vi "IMMU - Get Gyro Offsets.vi"(8 "error in (no error)":errorcluster, 11 "I2C Ref In":T1={"myRIO Reference"={"myRIO Model"=enum."Unknown", "myRIO Hardware Reference"={"Generic FPGA Reference"=refnum, "Allow multiple opens"=FALSE}}, "I2C Channels Enum"=enum."Not Connected", "I2C Configuration"={"I2C Transfer Rate"=enum."Fast mode (400 kbps)"}}) -> (0 "error out":errorcluster, 2 "Output Offset Array (int)":i16[](array[numeric]), 3 "I2C Ref Out":T1={"myRIO Reference"={"myRIO Model"=enum."Unknown", "myRIO Hardware Reference"={"Generic FPGA Reference"=refnum, "Allow multiple opens"=FALSE}}, "I2C Channels Enum"=enum."Not Connected", "I2C Configuration"={"I2C Transfer Rate"=enum."Fast mode (400 kbps)"}})   [LabVIEW 2021]
uses:
  <vilib>/myRIO/Instrument Drivers/Onboard IO/I2C/typedefs/I2C Reference.ctl
  <vilib>/myRIO/Common/Instrument Driver Framework/Utilities/typedefs/myRIO Generic Hardware Reference.ctl
  <vilib>/myRIO/Common/Instrument Driver Framework/Utilities/typedefs/Hardware Version Enum.ctl
  <vilib>/myRIO/Common/Instrument Driver Framework/Utilities/typedefs/myRIO v1.0 Reference.ctl
  <vilib>/myRIO/Common/Instrument Driver Framework/Utilities/typedefs/Generic FPGA Reference.ctl
  <vilib>/myRIO/Common/Instrument Driver Framework/myRIO v1.0/I2C/typedefs/I2C Channels Enum.ctl
  <vilib>/myRIO/Instrument Drivers/Onboard IO/I2C/typedefs/I2C Configuration.ctl
  <vilib>/myRIO/Instrument Drivers/Onboard IO/I2C/typedefs/I2C Transfer Rate.ctl
  <vilib>/Platform/TimedLoop/XDataNode/timing_clust.ctl
  <vilib>/Platform/TimedLoop/XDataNode/nitl_modes.ctl
  <vilib>/Platform/TimedLoop/XDataNode/wakeup.ctl
  <vilib>/Utility/error.llb/Error Cluster From Error Code.vi
  <vilib>/myRIO/Common/Instrument Driver Framework/myRIO v1.0/I2C/vis/myRIO v1.0 Write I2C.vi
  <vilib>/myRIO/Common/Instrument Driver Framework/myRIO v1.0/I2C/vis/myRIO v1.0 Read I2C.vi
  <vilib>/platform/TimedLoop/XDataNode/XDataNode.xnode
  <vilib>/Platform/TimedLoop/XDataNode/XDNodeRunTimeDep.lvlib
  <vilib>/myRIO/Instrument Drivers/Onboard IO/I2C/I2C.lvlib
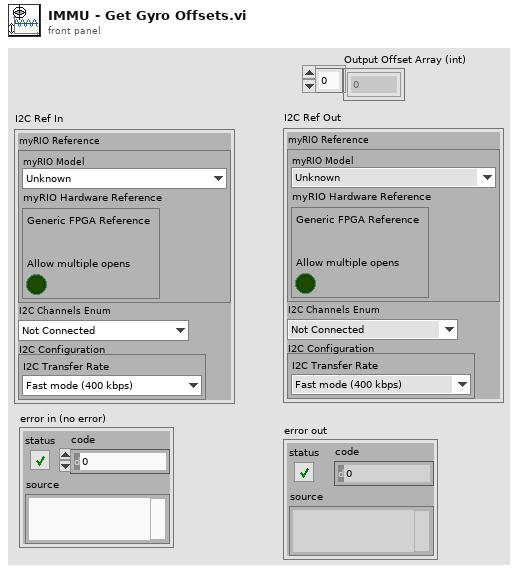
[diagram p1: front panel]
types:
  T1 = typedef "I2C.lvlib/I2C Reference.ctl" = cluster{"myRIO Reference":T2, "I2C Channels Enum":T6, "I2C Configuration":T7}
  T2 = typedef "myRIO Generic Hardware Reference.ctl" = cluster{"myRIO Model":T3, "myRIO Hardware Reference":T4}
  T3 = typedef "Hardware Version Enum.ctl" = enum16{"Unknown", "myRIO-1900", "myRIO-1950", "roboRIO", "NI ELVIS RIO CM", "ELVIS III"}
  T4 = typedef "myRIO v1.0 Reference.ctl" = cluster{"Generic FPGA Reference":T5, "Allow multiple opens":bool}
  T5 = typedef "Generic FPGA Reference.ctl" = refnum<k20>
  T6 = typedef "I2C Channels Enum.ctl" = enum16{"Not Connected", "A/I2C", "B/I2C", "I2C/I2C"}
  T7 = typedef "I2C.lvlib/I2C Configuration.ctl" = cluster{"I2C Transfer Rate":T8}
  T8 = typedef "I2C.lvlib/I2C Transfer Rate.ctl" = enum16{"Standard mode (100 kbps)", "Fast mode (400 kbps)"}
  T9 = typedef "XDNodeRunTimeDep.lvlib/timing_clust.ctl" = cluster{"Expected End [f-1]":u64, "Actual End [f-1]":u64, "Finished Late? [f-1]":bool, "Expected End [i-1]":u64, "Actual End [i-1]":u64, "Finished Late? [i-1]":bool, "Expected Start [i]":u64, "Actual Start [i]":u64, "Expected Start [f]":u64, "Actual Start [f]":u64, "Source Name":string, "Structure Name":string, "Period":i64, "Deadline":i64, "Offset":i64, "Start":i64, "Priority":i32, "Timeout":i32, "Mode":T10, "Wakeup Reason":T11, "Error":errorcluster, "Source Type":string, "Secondary Source Type":string, "Global End Time":u64, "Global Start Time":u64, "Frame Duration":u64, "Iteration Duration":u64, "Assigned CPU":i32, "I/O Scan Engine Mode":u32}
  T10 = typedef "XDNodeRunTimeDep.lvlib/nitl_modes.ctl" = enum32{"No Change", "Process missed periods, maintain original phase", "Discard missed periods, maintain original phase", "Process missed periods, ignore original phase", "Discard missed periods, ignore original phase"}
  T11 = typedef "XDNodeRunTimeDep.lvlib/wakeup.ctl" = enum32{"Normal", "Aborted", "Asynchronous wakeup", "Timing source error", "Timed loop error", "Timeout"}
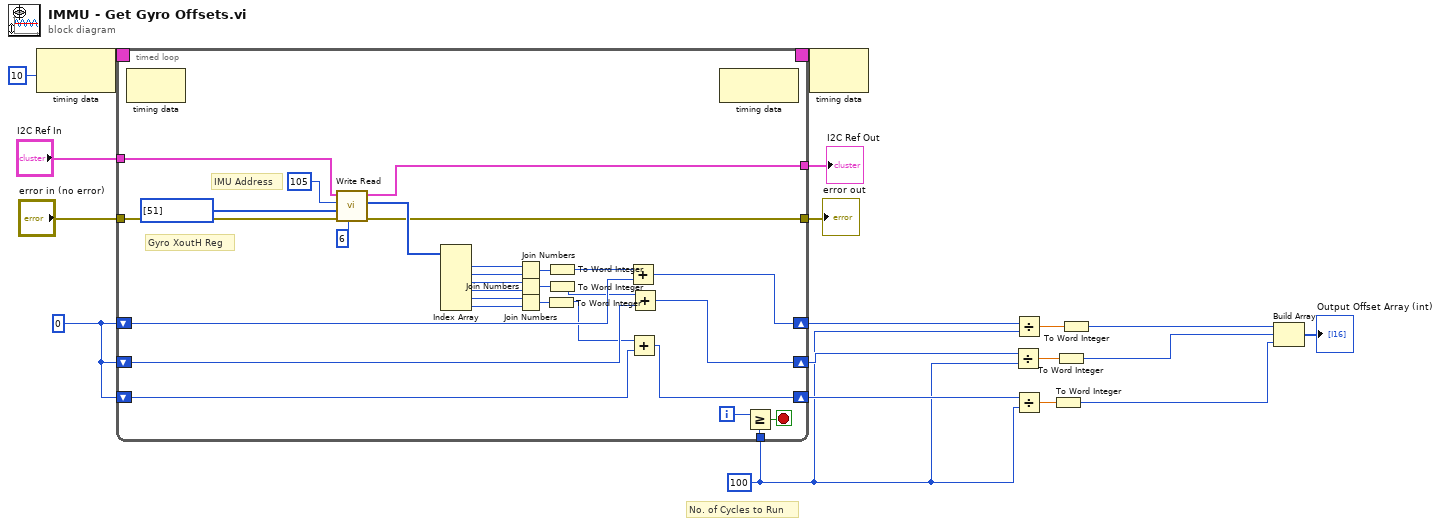
[diagram p0: block diagram]
diagram:
  w4 = 100 ("y")
  w12 = 0
  # "No. of Cycles to Run"
  n1 = node-c288(i64 10 ("Period")) -> (w19:T9)
  n2 = timed-loop {
    timing: w19 -> [_]
    timing-out: [_] -> w18
    shift-right: [w39] -> w17
    shift-left: w12 -> [w40]
    shift-right: [w37] -> w16
    shift-left: w12 -> [w38]
    shift-right: [w35] -> w15
    shift-left: w12 -> [w36]
    tunnel: "error in (no error)" -> [w26]
    tunnel: w4 -> [w28]
    tunnel: "I2C Ref In" -> [w22]
    tunnel: [w21] -> w2
    tunnel: [w20] -> w1
    i -> [w47]
    stop <- w46 stop-if-true
    # "Gyro XoutH Reg"
    # "IMU Address"
    n3 = node-c288() -> ()  [unwired: 1 in, 1 out]
    n4 = call <vilib>:"Write Read.vi"("Byte Count"=u32 6, "error in (no error)"=w26, "Bytes to Write"=u8[] [51], "Slave Address (7-bit)"=u8 105, "I2C Ref In"=w22) -> ("error out"=w21:errorcluster, "Bytes Read"=w27:u8[], "I2C Ref Out"=w20:T1)  [unwired: 3 in]
    n5 = Index Array(array=w27) -> (element #1=w48:u8, element #2=w45:u8, element #3=w44:u8, element #4=w43:u8, element #5=w42:u8, element #6=w41:u8)  [unwired: 6 in]
    n6 = Join Numbers(hi=w48, lo=w45) -> ((hi.lo)=w30:u16)
    n7 = Join Numbers(hi=w44, lo=w43) -> ((hi.lo)=w31:u16)
    n8 = Join Numbers(hi=w42, lo=w41) -> ((hi.lo)=w34:u16)
    n9 = To Word Integer(number=w34) -> (16bit integer=w33:i16)
    n10 = To Word Integer(number=w30) -> (16bit integer=w29:i16)
    n11 = To Word Integer(number=w31) -> (16bit integer=w32:i16)
    n12 = Add(x=w29, y=w40) -> (x+y=w39:i32)
    n13 = Add(x=w33, y=w36) -> (x+y=w35:i32)
    n14 = Add(x=w32, y=w38) -> (x+y=w37:i32)
    n15 = node-c288() -> ()  [unwired: 1 in, 1 out]
    n16 = Greater Or Equal?(x=w47, y=w28) -> (x >= y?=w46:bool)
  }
  "error out" <- w2
  "I2C Ref Out" <- w1
  n17 = node-c288(w18) -> ()  [unwired: 1 out]
  n18 = Divide(x=w16, y=w4) -> (x/y=w9:dbl)
  n19 = Divide(x=w17, y=w4) -> (x/y=w10:dbl)
  n20 = Divide(x=w15, y=w4) -> (x/y=w8:dbl)
  n21 = To Word Integer(number=w8) -> (16bit integer=w7:i16)
  n22 = To Word Integer(number=w9) -> (16bit integer=w6:i16)
  n23 = To Word Integer(number=w10) -> (16bit integer=w5:i16)
  n24 = Build Array(w5, w6, w7) -> (→"Output Offset Array (int)":i16[])
